vi "Send Configure FM Internal [FM].vi"(6 "modulation frequency (1000 Hz)":dbl[unit]=1000.0 format="%^.2e", 7 "Message Priority (Normal)":T1=enum."Normal", 8 "error in (no error)":errorcluster, 9 "peak deviation (100 Hz)":dbl[unit]=100.0 format="%^.2e", 10 "modulation waveform (Sine)":i32(ring)=1 items=["Sine"=1, "Square"=2, "Triangle"=3, "Ramp Up"=4, "Ramp Down"=5], 11 "Message Enqueuer":refnum<class "Message Enqueuer.lvclass">) -> (0 "error out":errorcluster, 3 "Message Enqueuer out":refnum<class "Message Enqueuer.lvclass">)   [LabVIEW 2013, in "CS++Fgen.lvlib" / "Configure FM Internal [FM] Msg.lvclass"]
doc: "This VI sends the message to an actor."
uses:
  Configure FM Internal [FM] Msg.lvclass
  <vilib>/ActorFramework/Message Enqueuer/Message Enqueuer.lvclass
  <vilib>/ActorFramework/Message Enqueuer/Message Priority.ctl
  Configure FM Internal [FM] Msg.lvclass/Configure FM Internal [FM] Msg.ctl
  <vilib>/ActorFramework/Message Enqueuer/Message Enqueuer.lvclass/Message Enqueuer.ctl
  <vilib>/ActorFramework/Message Priority Queue/Priority Enqueue.vi
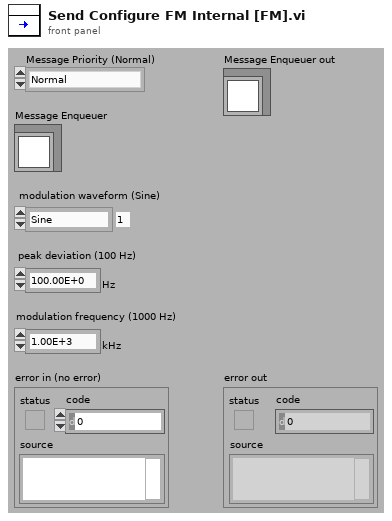
[diagram p1: front panel]
types:
  T1 = typedef "Actor Framework.lvlib/Message Enqueuer.lvclass/Message Priority.ctl" = enum16{"Low", "Normal", "High"}
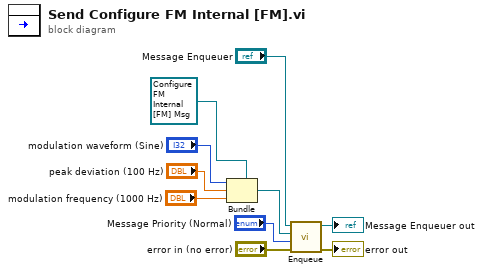
[diagram p0: block diagram]
diagram:
  n1 = Bundle(cluster=refnum<class "Configure FM Internal [FM] Msg.lvclass"> refnum ("Object"), "modulation waveform (Sine)", "peak deviation (100 Hz)", "modulation frequency (1000 Hz)") -> (w6:refnum<class "Configure FM Internal [FM] Msg.lvclass">)
  n2 = call <vilib>:"Enqueue.vi"("error in (no error)"="error in (no error)", "Message Priority (Normal)"="Message Priority (Normal)", "Message"=w6, "Message Enqueuer in"="Message Enqueuer") -> ("error out"=→"error out":errorcluster, "Message Enqueuer out"=→"Message Enqueuer out":refnum<class "Message Enqueuer.lvclass">)  [unwired: 6 in]
